vi "init.vi"(8 "error in (no error)":errorcluster, 11 "Logger in":refnum<class "TestDataLog.lvclass">) -> (0 "error out":errorcluster, 3 "Logger out":refnum<class "TestDataLog.lvclass">)   [LabVIEW 2013, in "TestDataLog.lvclass"]
uses:
  TestDataLog.lvclass
  <userlib>/Common/Log/Config/Log.ctl
  Configuration/TestParameters.ctl
  Configuration/CycleProfileConfig.ctl
  TestDataLog.lvclass/TestDataLog.ctl
  <userlib>/Common/Log/Log/Log.lvclass/Log.ctl
  ConfigurationThisComponent/ConfigurationThisComponent.lvclass
  <userlib>/Common/Log/Log/Log.lvclass
  <userlib>/Common/Log/Log.lvlib
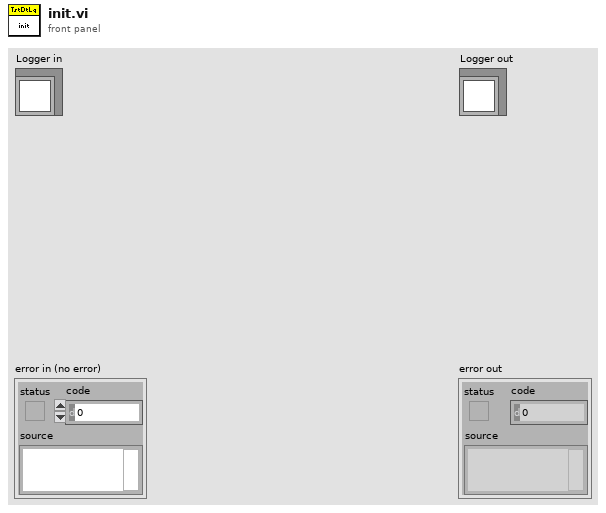
[diagram p1: front panel]
types:
  T1 = typedef "TestParameters.ctl" = cluster{"Number of cycles for complete test":u32, "Cycle profile":T2, "PGA Gain Coefficients":u8[], "Temperature Transition Wait Time":dbl[unit], "Temperature Settled StDev":dbl[unit], "Temperature Settling Sample Size":u16, "Bridge Measurement Sample Size":u16}
  T2 = typedef "CycleProfileConfig.ctl" = cluster{"Temperature Setpoint":dbl[unit][], "Soak Time":dbl[unit][], "Gain Stabilization Time":dbl[unit][], "Pause After Step":dbl[unit][]}
  T3 = typedef "Log.lvlib/Log.ctl" = cluster{"Log Directory":path, "Log Filename Base":string, "Max records per file":u32, "Comment":string}
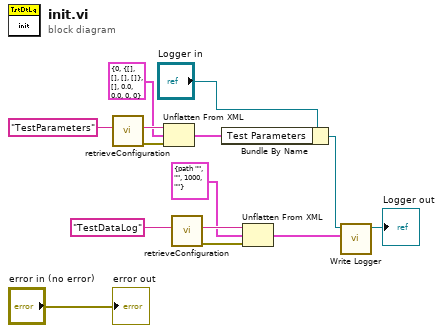
[diagram p0: block diagram]
diagram:
  n1 = call "retrieveConfiguration.vi"("configName"="TestParameters") -> ("error out"=w5:errorcluster, "xmlConfig"=w4:string)  [unwired: 8 in, 1 out]
  n2 = Unflatten From XML(xml string=w4, type=T1 {"Number of cycles for complete test"=0, "Cycle profile"={"Temperature Setpoint"=[], "Soak Time"=[], "Gain Stabilization Time"=[], "Pause After Step"=[]}, "PGA Gain Coefficients"=[], "Temperature Transition Wait Time"=0.0, "Temperature Settled StDev"=0.0, "Temperature Settling Sample Size"=0, "Bridge Measurement Sample Size"=0} ("Test Parameters"), error in (no error)=w5) -> (value=w2:T1)  [unwired: 1 out]
  n3 = call "retrieveConfiguration.vi"("configName"="TestDataLog") -> ("error out"=w11:errorcluster, "xmlConfig"=w12:string)  [unwired: 8 in, 1 out]
  n4 = Bundle By Name(cluster="Logger in", "Test Parameters"=w2) -> (w9:refnum<class "TestDataLog.lvclass">)
  n5 = Unflatten From XML(xml string=w12, type=T3 {"Log Directory"=path "", "Log Filename Base"="", "Max records per file"=1000, "Comment"=""} ("Logger"), error in (no error)=w11) -> (value=w7:T3)  [unwired: 1 out]
  n6 = call <userlib>:"Write Logger.vi"("Logger"=w7, "Logger in"=w9) -> ("Logger out"=→"Logger out":refnum<class "TestDataLog.lvclass">)  [unwired: 9 in]
  "error out" <- "error in (no error)"
